vi "Single Z Ramp Waveforms.vi"(1 "Second Phase Offset":dbl, 2 "Initial Phase Offset":dbl) -> (0 "Output Waveforms":waveform(dbl)[](array[waveform]))   [LabVIEW 2013]
uses:
  <vilib>/Waveform/WDTOps.llb/WDT Append Waveforms DBL.vi
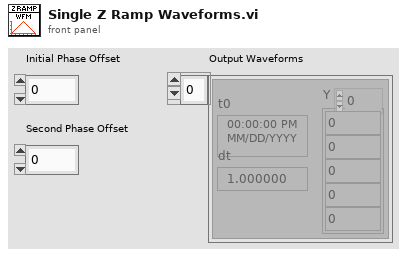
[diagram p1: front panel]
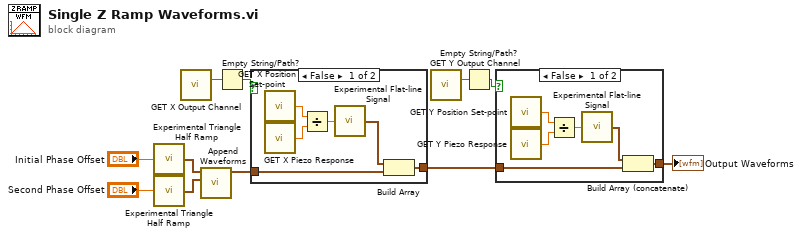
[diagram p0: block diagram]
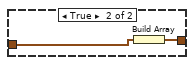
[diagram p3: hidden frame]
diagram:
  n1 = call "Experimental Triangle Half Ramp.vi"("Phase Offset"="Initial Phase Offset") -> ("Half Triangle"=w10:waveform(dbl))
  n2 = call "Experimental Triangle Half Ramp.vi"("Phase Offset"="Second Phase Offset") -> ("Half Triangle"=w7:waveform(dbl))
  n3 = call "GET X Output Channel.vi"() -> ("X Output Channel"=w4:string)
  n4 = call-poly <vilib>:"Append Waveforms.vi"("waveform B"=w7, "waveform A"=w10) -> ("waveform out"=w11:waveform(dbl))  [unwired: 8 in, 1 out]
  n5 = Empty String/Path?(string/path=w4) -> (empty?=w3:bool)
  n6 = case shown="False" w3 {
    tunnel: w11 -> [w14 w18]
    tunnel: [w12 w19] -> w2
    frame False {
      n7 = call "GET X Position Set-point.vi"() -> ("X Position Set-point"=w16:dbl)
      n8 = call "GET X Piezo Response.vi"() -> ("X Piezo Response"=w17:dbl)
      n9 = Divide(x=w16, y=w17) -> (x/y=w15:dbl)
      n10 = call "Experimental Flat-line Signal.vi"("Flatline Offset"=w15) -> ("Flatline Signal"=w13:waveform(dbl))
      n11 = Build Array(w13, w14) -> (w12:waveform(dbl)[])
    }
    frame True {
      n12 = Build Array(w18) -> (w19:waveform(dbl)[])
    }
  }
  n13 = call "GET Y Output Channel.vi"() -> ("Y Output Channel"=w6:string)
  n14 = Empty String/Path?(string/path=w6) -> (empty?=w5:bool)
  n15 = case shown="False" w5 {
    tunnel: w2 -> [w22 w26]
    tunnel: [w20 w26] -> w1
    frame False {
      n16 = call "GET Y Position Set-point.vi"() -> ("Y Position Set-point"=w24:dbl)
      n17 = call "GET Y Piezo Response.vi"() -> ("Y Piezo Response"=w25:dbl)
      n18 = Divide(x=w24, y=w25) -> (x/y=w23:dbl)
      n19 = call "Experimental Flat-line Signal.vi"("Flatline Offset"=w23) -> ("Flatline Signal"=w21:waveform(dbl))
      n20 = Build Array (concatenate)(w21, w22) -> (w20:waveform(dbl)[])
    }
    frame True {
    }
  }
  "Output Waveforms" <- w1
